vi "Card Input Ref.vi"(7 "Action":enum16{"Initial", "Write", "Read", "Release"}(ring)=enum."Release", 8 "error In":errorcluster, 10 "CardIndex":i32, 11 "RefIn":refnum<vi>) -> (0 "error Out":errorcluster, 3 "RefOut":refnum<vi>)   [LabVIEW 2019, in "IOCard.lvclass"]
uses:
  IOCard.lvclass
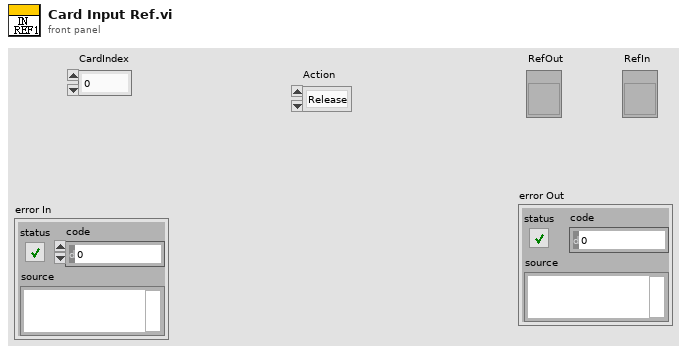
[diagram p1: front panel]
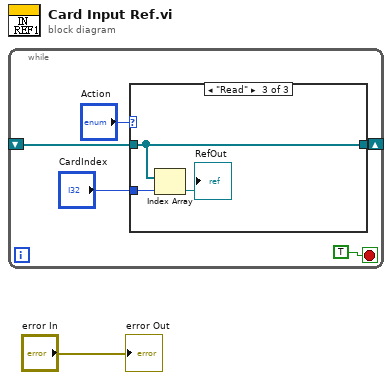
[diagram p0: block diagram]
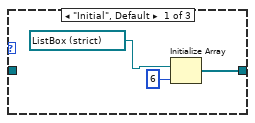
[diagram p2: hidden frame]
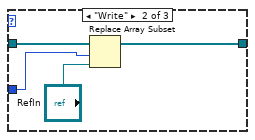
[diagram p3: hidden frame]
diagram:
  n1 = while {
    shift-right: [w4] -> _
    shift-left: _ -> [w3]
    stop <- TRUE stop-if-true
    n2 = case shown="\"Read\"" "Action" {
      tunnel: [w8 w12 w15] -> w4
      tunnel: w3 -> [_ w13 w15]
      tunnel: "CardIndex" -> [_ w11 w16]
      frame "Initial", Default {
        n3 = Initialize Array(refnum<vi> refnum ("Lst_Output 2"), 6 ("dimension size")) -> (w8:refnum<vi>[])
      }
      frame "Write" {
        n4 = Replace Array Subset(array=w13, new element="RefIn", index=w11) -> (w12:refnum<vi>[])
      }
      frame "Read" {
        n5 = Index Array(array=w15, index=w16) -> (element=→"RefOut":refnum<vi>)
      }
    }
  }
  "error Out" <- "error In"
